vi "Remove Session (byClientID).vi"(8 "error in (no error)":errorcluster, 10 "Client ID":string, 11 "MQTT Server":refnum<class "Server.lvclass">) -> (0 "error out":errorcluster, 1 "removed":bool, 2 "Client ID dup":string, 3 "MQTT Server":refnum<class "Server.lvclass">, 5 "SessionMailbox":refnum<queue>)   [LabVIEW 2013, in "MQTT Server.lvlib" / "Server.lvclass"]
uses:
  Server.lvclass
  <vilib>/LabVIEW Open Source Project/MQTT Connection/MQTT_Base/Base Class/Response -- cluster.ctl
  <vilib>/LabVIEW Open Source Project/MQTT Control Packets/Control Packets/ControlPacket/ControlPacket.lvclass
  Server.lvclass/Server.ctl
  <vilib>/LabVIEW Open Source Project/MQTT Connection/MQTT_Base/Base Class/MQTT_Base.lvclass
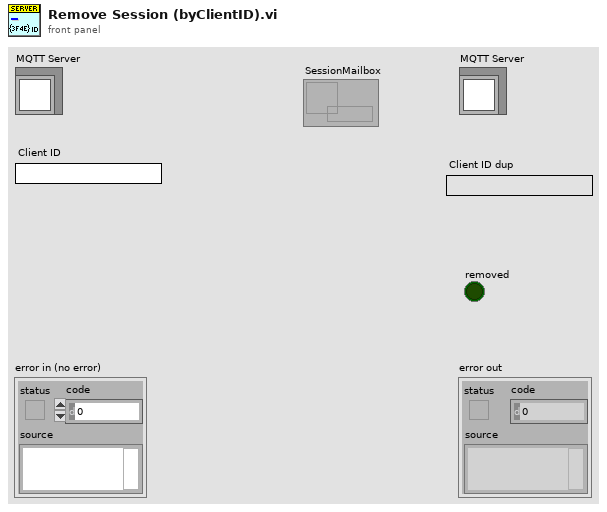
[diagram p1: front panel]
types:
  T1 = typedef "MQTT Server.lvlib/Server.lvclass/SessionRef -- cluster.ctl" = cluster{"ClientID":string, "SessionMailbox":refnum<queue>}
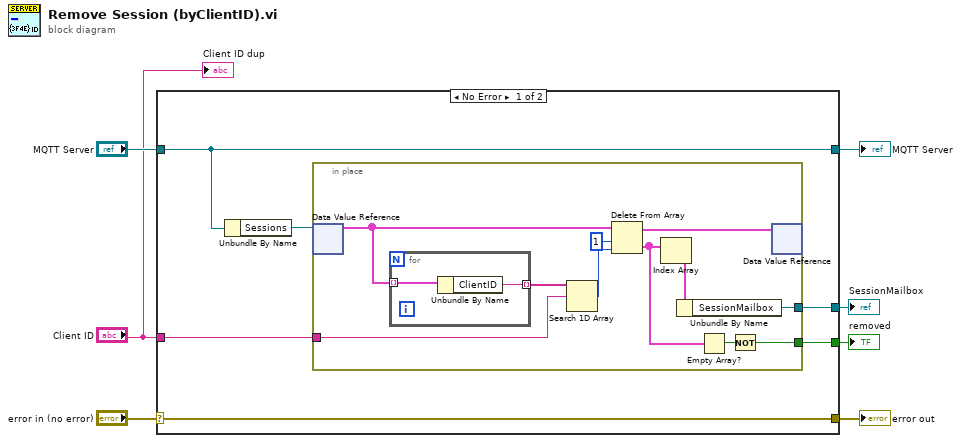
[diagram p0: block diagram]
diagram:
  n1 = case shown="No Error" "error in (no error)" {
    selector: "error in (no error)" -> [w10 w28]
    tunnel: [w10 w28] -> w6
    tunnel: [w12 w27] -> w4
    tunnel: "MQTT Server" -> [w12 w27]
    tunnel: "Client ID" -> [w11 _]
    tunnel: [w9 _] -> w2
    tunnel: [w8 _] -> w1
    frame No Error {
      n2 = Unbundle By Name(w12) -> ("Sessions"=w13:refnum<data-value>)
      n3 = in-place {
        in-place-border: w11 -> [w23]
        in-place-border: [w17] -> w9
        in-place-border: [w14] -> w8
        n4 = in-place-dvr #1(w13) -> (w22:T1[])  [unwired: 1 out]
        n5 = for {
          tunnel: w22 -> [w26] mode=indexing
          tunnel: [w25] -> w24 mode=indexing
          n6 = Unbundle By Name(w26) -> ("ClientID"=w25:string)
        }
        n7 = Search 1D Array(1D array=w24, element=w23) -> (index of element=w20:i32)  [unwired: 1 in]
        n8 = Delete From Array(array=w22, length=1, index=w20) -> (deleted portion=w16:T1[], array with subset deleted=w19:T1[])
        n9 = Index Array(array=w16) -> (element=w18:T1)  [unwired: 1 in]
        n10 = Unbundle By Name(w18) -> ("SessionMailbox"=w17:refnum<queue>)
        n11 = Empty Array?(array=w16) -> (empty?=w15:bool)
        n12 = Not(x=w15) -> (.not. x?=w14:bool)
        n13 = in-place-dvr #1(w19) -> ()  [unwired: 2 out]
      }
    }
    frame Error {
    }
  }
  "error out" <- w6
  "MQTT Server" <- w4
  "SessionMailbox" <- w2
  "removed" <- w1
  "Client ID dup" <- "Client ID"
